vi "front_panel.vi"() -> ()   [LabVIEW 2017]
uses:
  controls/Left Menu.ctl
  controls/Right Menu.ctl
  controls/ConsumerCtl.ctl
  controls/ConsumerCmd.ctl
  controls/DisplayCmd.ctl
  controls/DisplayCtl.ctl
  controls/EnableDisableCmd.ctl
  controls/UpdateMessageCtl.ctl
  controls/UpdateMessageCmd.ctl
  controls/UpdateMenuCmd.ctl
  controls/ElapsedTimeCmd.ctl
panel:
  out "Right Menu":T1
  in  "Reset Button":bool
  in  "Stop Button":bool
  in  "Enter Button":bool
  in  "Start Button":bool
  in  "User Input":string
  out "Box5":bool
  out "Box4":bool
  out "Box3":bool
  out "Box2":bool
  out "Box1":bool
  in  "Right Buttons":cluster{"Button 3":bool, "Button 4":bool}
  in  "Left Buttons":cluster{"Button 1":bool, "Button 2":bool}
  out "Screen":string
  out "Left Menu":T2
  # "Parcel Locker"
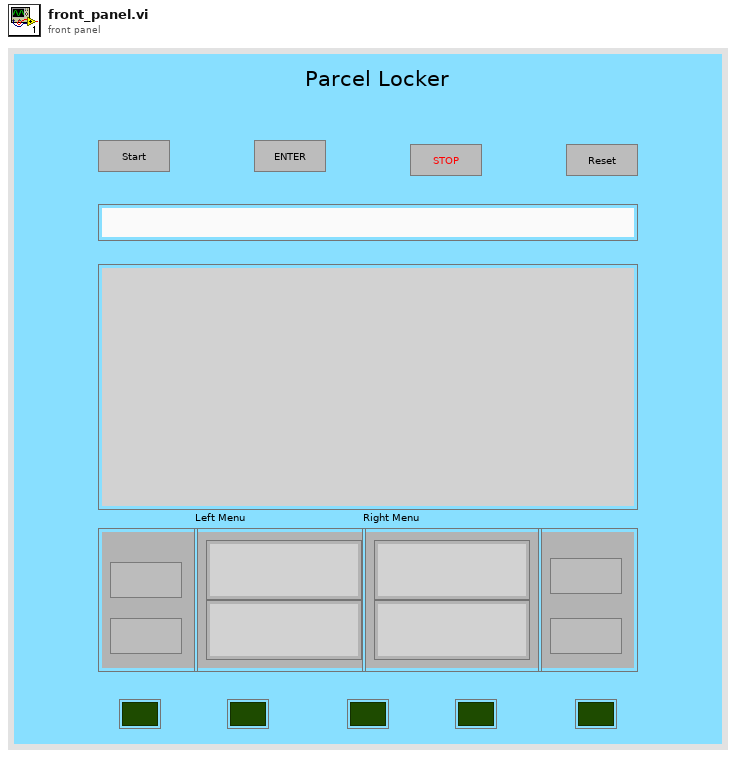
[diagram p1: front panel]
types:
  T1 = typedef "Left Menu.ctl" = cluster{"Indicator1":string, "Indicator4":string}
  T2 = typedef "Right Menu.ctl" = cluster{"Indicator1":string, "Indicator4":string}
  T3 = typedef "DisplayCmd.ctl" = cluster{"Command":T4, "Data":variant}
  T4 = typedef "DisplayCtl.ctl" = enum16{"Initialize", "Enable/Disable Controls", "FocusCursor", "UpdateMessage", "Update Menus", "Finish Operation", "Exit", "Clean User Input"}
  T5 = typedef "ConsumerCtl.ctl" = cluster{"Command":T6, "Data":variant}
  T6 = typedef "ConsumerCmd.ctl" = enum16{"User Input", "Left Button", "Right Button", "Exit", "Start operation", "Initialize"}
  T7 = typedef "EnableDisableCmd.ctl" = enum16{"InitialSetup", "Disable Menus", "Enable Menus", "Disable User Input", "Enable User Input"}
  T8 = enum8{"Enabled", "Disabled", "Disabled and Grayed Out"}[]
  T9 = typedef "UpdateMessageCtl.ctl" = cluster{"Command":T10, "Data":variant}
  T10 = typedef "UpdateMessageCmd.ctl" = enum16{"Welcome", "Main Menu", "Account Failed", "Session Terminated", "Deposit", "Deposit Complete", "Withdrawal", "Withdrawal Complete"}
  T11 = typedef "UpdateMenuCmd.ctl" = enum16{"NoMenu", "MainMenu"}
  T12 = typedef "ElapsedTimeCmd.ctl" = enum16{"Start", "Stop", "Check Time"}
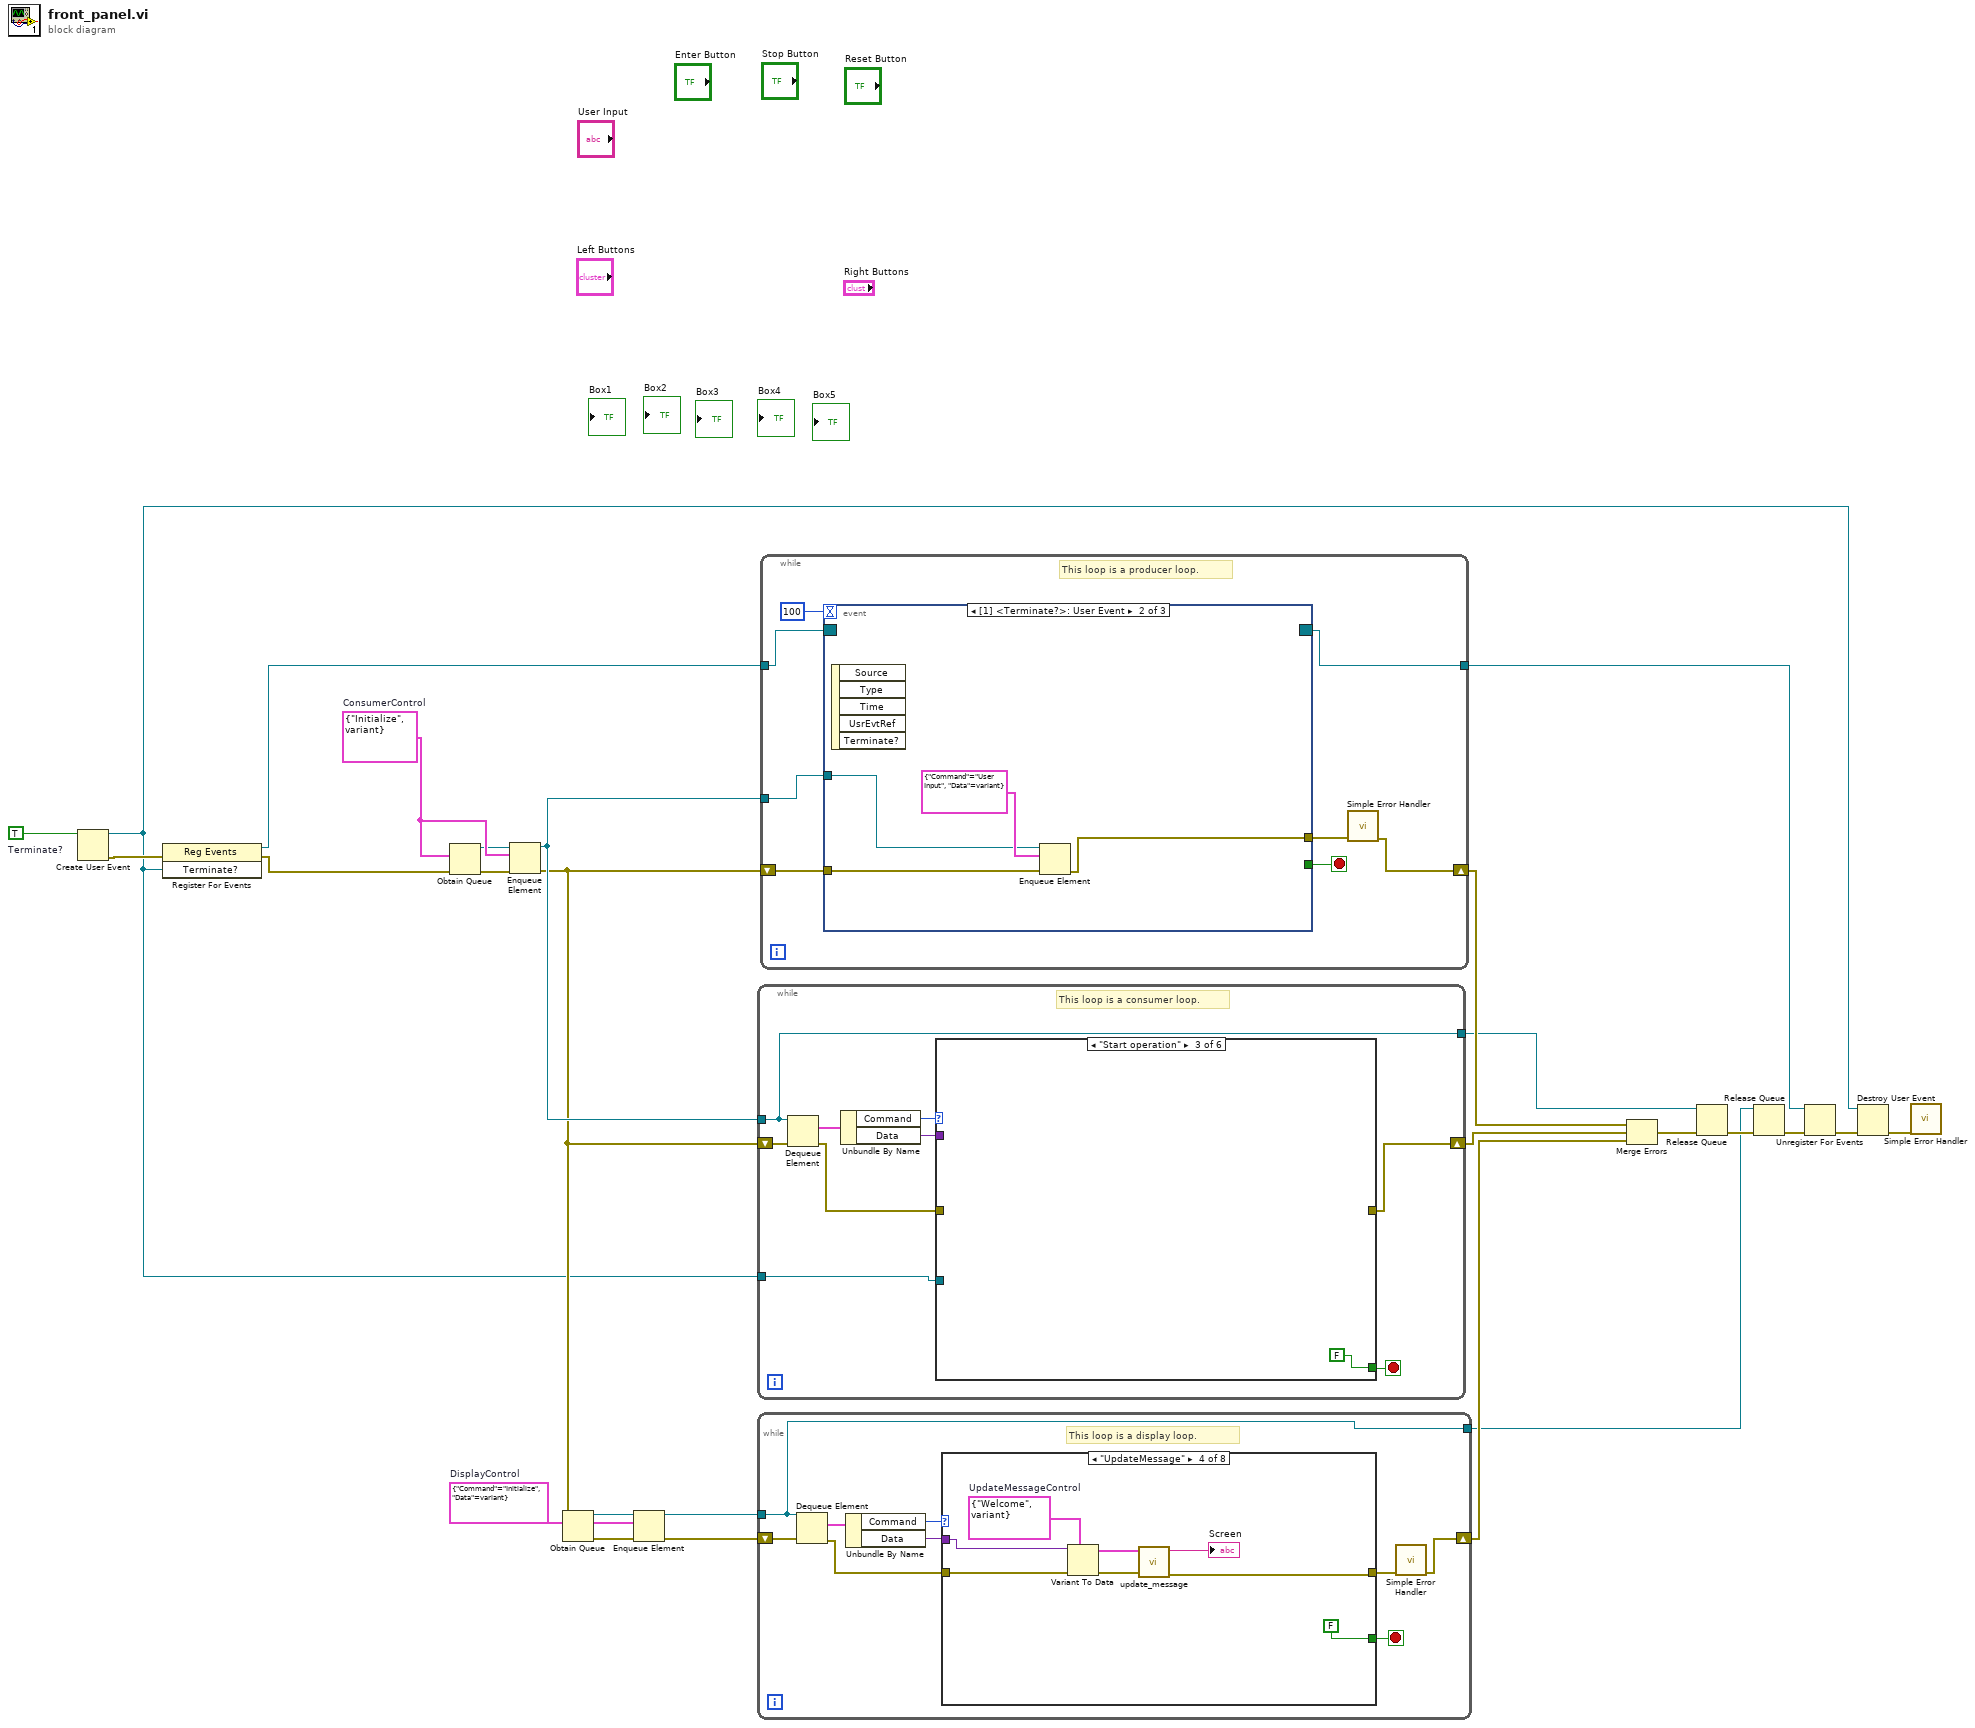
[diagram p0: block diagram]
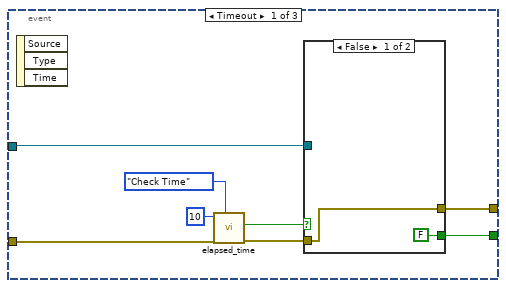
[diagram p2: hidden frame]
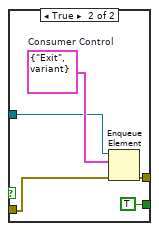
[diagram p3: hidden frame]
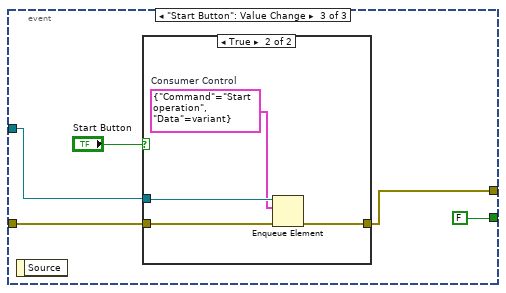
[diagram p4: hidden frame]
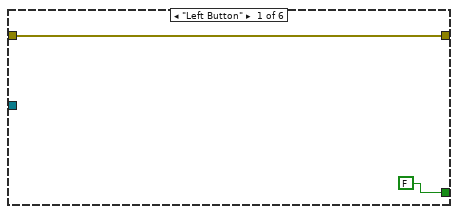
[diagram p6: hidden frame]
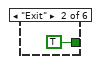
[diagram p7: hidden frame]
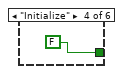
[diagram p8: hidden frame]
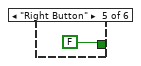
[diagram p9: hidden frame]
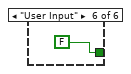
[diagram p10: hidden frame]
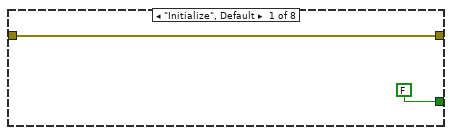
[diagram p11: hidden frame]
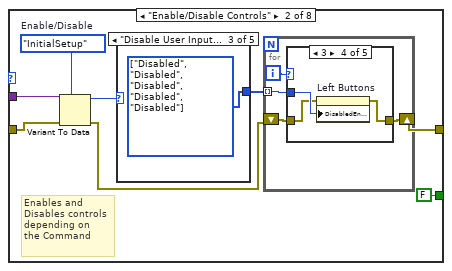
[diagram p12: hidden frame]
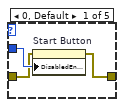
[diagram p13: hidden frame]
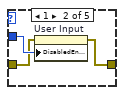
[diagram p14: hidden frame]
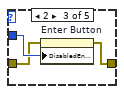
[diagram p15: hidden frame]
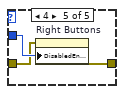
[diagram p16: hidden frame]
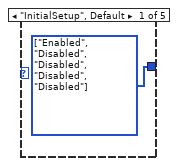
[diagram p17: hidden frame]
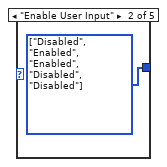
[diagram p18: hidden frame]
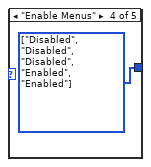
[diagram p19: hidden frame]
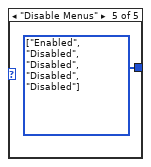
[diagram p20: hidden frame]
diagram:
  w8 = TRUE  # Terminate?
  w22 = T3 {"Command"=enum."Initialize", "Data"=variant}  # DisplayControl
  w14 = T5 {"Command"=enum."Initialize", "Data"=variant}  # ConsumerControl
  n1 = Create User Event(user event datatype=w8) -> (user event=w3:refnum<user-event>, error out=w4:errorcluster)  [unwired: 1 in]
  n2 = register-events(error in=w4, w3) -> (reference out=w2:refnum<event-registration>, error out=w1:errorcluster)  [unwired: 1 in]
  n3 = Obtain Queue(element data type=w14, error in (no error)=w1) -> (queue out=w13:refnum<queue>, error out=w11:errorcluster)  [unwired: 3 in, 1 out]
  n4 = Enqueue Element(queue=w13, element=w14, error in (no error)=w11) -> (queue out=w12:refnum<queue>, error out=w10:errorcluster)  [unwired: 1 in, 1 out]
  n5 = Obtain Queue(element data type=w22, error in (no error)=w10) -> (queue out=w26:refnum<queue>, error out=w24:errorcluster)  [unwired: 3 in, 1 out]
  n6 = Enqueue Element(queue=w26, element=w22, error in (no error)=w24) -> (queue out=w25:refnum<queue>, error out=w23:errorcluster)  [unwired: 1 in, 1 out]
  n7 = while {
    shift-right: [w30] -> w20
    shift-left: w10 -> [w32]
    tunnel: w12 -> [w27]
    tunnel: w3 -> [w28]
    tunnel: [w27] -> w5
    stop <- w29 stop-if-true
    # "This loop is a consumer loop."
    n8 = Dequeue Element(queue=w27, error in (no error)=w32) -> (element=w35:T5, error out=w31:errorcluster)  [unwired: 1 in, 2 out]
    n9 = Unbundle By Name(w35) -> ("Command"=w34:T6, "Data"=w33:variant)
    n10 = case shown="\"Start operation\"" w34 {
      tunnel: w33 -> [_ _ _ _ _ _]
      tunnel: w31 -> [w37 _ _ _ _ _]
      tunnel: [w37 _ _ _ _ _] -> w30
      tunnel: [FALSE TRUE ("Start Button") FALSE FALSE FALSE FALSE] -> w29
      tunnel: w28 -> [_ _ _ _ _ _]
      frame "Left Button" {
      }
      frame "Exit" {
      }
      frame "Start operation" {
      }
      frame "Initialize" {
      }
      frame "Right Button" {
      }
      frame "User Input" {
      }
    }
  }
  n11 = while {
    tunnel: w25 -> [w43]
    shift-right: [w45] -> w21
    shift-left: w23 -> [w51]
    tunnel: [w43] -> w6
    stop <- w44 stop-if-true
    # "This loop is a display loop."
    n12 = Dequeue Element(queue=w43, error in (no error)=w51) -> (element=w50:T3, error out=w47:errorcluster)  [unwired: 1 in, 2 out]
    n13 = Unbundle By Name(w50) -> ("Command"=w49:T4, "Data"=w48:variant)
    n14 = case shown="\"UpdateMessage\"" w49 {
      tunnel: w48 -> [_ w60 _ w96 w104 _ _ _]
      tunnel: w47 -> [w53 w59 w87 w95 w105 w109 w111 w113]
      tunnel: [w53 w54 w86 w91 w100 w109 w111 w113] -> w46
      tunnel: [FALSE ("Start Button") FALSE ("Start Button") FALSE ("Start Button") FALSE ("Start Button") FALSE ("Start Button") FALSE ("Start Button") TRUE ("Start Button") FALSE ("Start Button")] -> w44
      frame "Initialize", Default {
      }
      frame "Enable/Disable Controls" {
        w56 = EnableDisableCmd."InitialSetup"  # Enable/Disable
        # "Enables and\nDisables controls\ndepending on\nthe Command"
        n15 = Variant To Data(error in=w59, type=w56, Variant=w60) -> (data=w57:T7, error out=w58:errorcluster)
        n16 = case shown="\"Disable User Input\"" w57 {
          tunnel: [w81 w82 w83 w84 w85] -> w55
          frame "InitialSetup", Default {
            w81 = T8 [enum."Enabled", enum."Disabled", enum."Disabled", enum."Disabled", enum."Disabled"] items=["Enabled", "Disabled", "Disabled and Grayed Out"]
          }
          frame "Enable User Input" {
            w82 = T8 [enum."Disabled", enum."Enabled", enum."Enabled", enum."Disabled", enum."Disabled"] items=["Enabled", "Disabled", "Disabled and Grayed Out"]
          }
          frame "Disable User Input" {
            w83 = T8 [enum."Disabled", enum."Disabled", enum."Disabled", enum."Disabled", enum."Disabled"] items=["Enabled", "Disabled", "Disabled and Grayed Out"]
          }
          frame "Enable Menus" {
            w84 = T8 [enum."Disabled", enum."Disabled", enum."Disabled", enum."Enabled", enum."Enabled"] items=["Enabled", "Disabled", "Disabled and Grayed Out"]
          }
          frame "Disable Menus" {
            w85 = T8 [enum."Enabled", enum."Disabled", enum."Disabled", enum."Disabled", enum."Disabled"] items=["Enabled", "Disabled", "Disabled and Grayed Out"]
          }
        }
        n17 = for {
          tunnel: w55 -> [w63] mode=indexing
          shift-right: [w62] -> w54
          shift-left: w58 -> [w65]
          i -> [w64]
          n18 = case shown="3" w64 {
            tunnel: w65 -> [w67 w70 w73 w76 w79]
            tunnel: w63 -> [w68 w71 w74 w77 w80]
            tunnel: [w66 w69 w72 w75 w78] -> w62
            frame 0, Default {
              n19 = property on="Start Button" class="Bool (strict)"(error in=w67, "DisabledEnum"=w68) -> (error out=w66:errorcluster)  [unwired: 1 in, 1 out]
            }
            frame 1 {
              n20 = property on="User Input" class="Str"(error in=w70, "DisabledEnum"=w71) -> (error out=w69:errorcluster)  [unwired: 1 in, 1 out]
            }
            frame 2 {
              n21 = property on="Enter Button" class="Bool"(error in=w73, "DisabledEnum"=w74) -> (error out=w72:errorcluster)  [unwired: 1 in, 1 out]
            }
            frame 3 {
              n22 = property on="Left Buttons" class="Clust"(error in=w76, "DisabledEnum"=w77) -> (error out=w75:errorcluster)  [unwired: 1 in, 1 out]
            }
            frame 4 {
              n23 = property on="Right Buttons" class="Clust"(error in=w79, "DisabledEnum"=w80) -> (error out=w78:errorcluster)  [unwired: 1 in, 1 out]
            }
          }
        }
      }
      frame "FocusCursor" {
        n24 = property on="User Input" class="Str"(error in=w87, "Key Focus"=TRUE) -> (error out=w86:errorcluster)  [unwired: 1 in, 1 out]
      }
      frame "UpdateMessage" {
        w94 = T9 {"Command"=enum."Welcome", "Data"=variant}  # UpdateMessageControl
        n25 = Variant To Data(error in=w95, type=w94, Variant=w96) -> (data=w93:T9, error out=w92:errorcluster)
        n26 = call "update_message.vi"("error in (no error)"=w92, "Cluster"=w93) -> ("error out"=w91:errorcluster, "Screen"=→"Screen":string)  [unwired: 7 in]
      }
      frame "Update Menus" {
        w103 = UpdateMenuCmd."MainMenu"  # UpdateMenuCommand
        n27 = Variant To Data(error in=w105, type=w103, Variant=w104) -> (data=w102:T11, error out=w101:errorcluster)
        n28 = call "update_menus.vi"("UpdateMenuCommand"=w102, "error in (no error)"=w101) -> ("error out"=w100:errorcluster, "Right Menu"=→"Right Menu":T1, "Left Menu"=→"Left Menu":T2)  [unwired: 7 in]
      }
      frame "Finish Operation" {
        n29 = local write "Start Button"(FALSE ("Start Button")) -> ()
      }
      frame "Exit" {
      }
      frame "Clean User Input" {
        n30 = local write "User Input"("") -> ()
      }
    }
    n31 = call <vilib>:"Simple Error Handler.vi"("error in (no error)"=w46) -> ("error out"=w45:errorcluster)  [unwired: 4 in, 4 out]
  }
  n32 = while {
    tunnel: w12 -> [w121]
    shift-right: [w118] -> w9
    shift-left: w10 -> [w120]
    tunnel: w2 -> [w116]
    tunnel: [w115] -> w7
    stop <- w117 stop-if-true
    # "This loop is a producer loop."
    n33 = event shown="[1] <Terminate?>: User Event" {
      selector: w116 -> [_ _ _]
      dyn-events: [_ _ _] -> w115
      timeout: 100 -> [_ _ _]
      tunnel: w121 -> [w130 w138 w142]
      tunnel: w120 -> [w125 w141 w146]
      tunnel: [w129 w140 w145] -> w119
      tunnel: [w128 _ FALSE] -> w117
      event Timeout {
        n34 = event-data() -> ()  [unwired: 1 in, 3 out]
        n35 = call "elapsed_time.vi"("Command"=ElapsedTimeCmd."Check Time", "error in (no error)"=w125, "Desired Time (s)"=u32 10) -> ("error out"=w126:errorcluster, "Is Done?"=w127:bool)  [unwired: 6 in, 1 out]
        n36 = case shown="False" w127 {
          tunnel: w130 -> [_ w135]
          tunnel: w126 -> [w131 w137]
          tunnel: [w131 w134] -> w129
          tunnel: [FALSE TRUE] -> w128
          frame False {
          }
          frame True {
            w136 = T5 {"Command"=enum."Exit", "Data"=variant}  # Consumer Control
            n37 = Enqueue Element(queue=w135, element=w136, error in (no error)=w137) -> (error out=w134:errorcluster)  [unwired: 1 in, 2 out]
          }
        }
      }
      event User Event {
        n38 = event-data() -> ()  [unwired: 1 in, 5 out]
        n39 = Enqueue Element(queue=w138, element=T5 {"Command"=enum."User Input", "Data"=variant} ("Cluster"), error in (no error)=w141) -> (error out=w140:errorcluster)  [unwired: 1 in, 2 out]
      }
      event "Start Button": Value Change {
        n40 = event-data() -> ()  [unwired: 1 in, 1 out]
        n41 = case shown="True" "Start Button" {
          tunnel: w146 -> [w147 w151]
          tunnel: [w147 w150] -> w145
          tunnel: w142 -> [_ w149]
          frame False {
          }
          frame True {
            w148 = T5 {"Command"=enum."Start operation", "Data"=variant}  # Consumer Control
            n42 = Enqueue Element(queue=w149, element=w148, error in (no error)=w151) -> (error out=w150:errorcluster)  [unwired: 1 in, 2 out]
          }
        }
      }
    }
    n43 = call <vilib>:"Simple Error Handler.vi"("error in (no error)"=w119) -> ("error out"=w118:errorcluster)  [unwired: 4 in, 4 out]
  }
  n44 = Merge Errors(w9, w20, w21) -> (w19:errorcluster)
  n45 = Release Queue(queue=w5, error in (no error)=w19) -> (error out=w18:errorcluster)  [unwired: 1 in, 2 out]
  n46 = Release Queue(queue=w6, error in (no error)=w18) -> (error out=w17:errorcluster)  [unwired: 1 in, 2 out]
  n47 = Unregister For Events(event registration refnum=w7, error in=w17) -> (error out=w16:errorcluster)
  n48 = Destroy User Event(user event=w3, error in=w16) -> (error out=w15:errorcluster)
  n49 = call <vilib>:"Simple Error Handler.vi"("error in (no error)"=w15) -> ()  [unwired: 4 in, 5 out]
